vi "Build_Header_ARG.vi"(9 "All_Bundled_Data_Brass":T1, 10 "ERD Number Array In":string[](array[string]), 11 "ERD Name Array In":string[](array[string])) -> (2 "ERD Name Array out 2":string[][](array[string]))   [LabVIEW 2021]
uses:
  Type defs/All_Bundled_Data_ARG.ctl
  Dryer Tool (Commercial 2)/JL Dryer Tool Support/type defs/Version.ctl
  Dryer Tool (Commercial 2)/JL Dryer Tool Support/type defs/CSV_File_String_Arrays.ctl
  Dryer Tool (Commercial 2)/JL Dryer Tool Support/type defs/Fault Table Array.ctl
  Dryer Tool (Commercial 2)/JL Dryer Tool Support/type defs/Fault_Table_Info.ctl
  Dryer Tool (Commercial 2)/JL Dryer Tool Support/type defs/BootloaderVersion.ctl
  Type defs/ERD_Always_Show_ARG.ctl
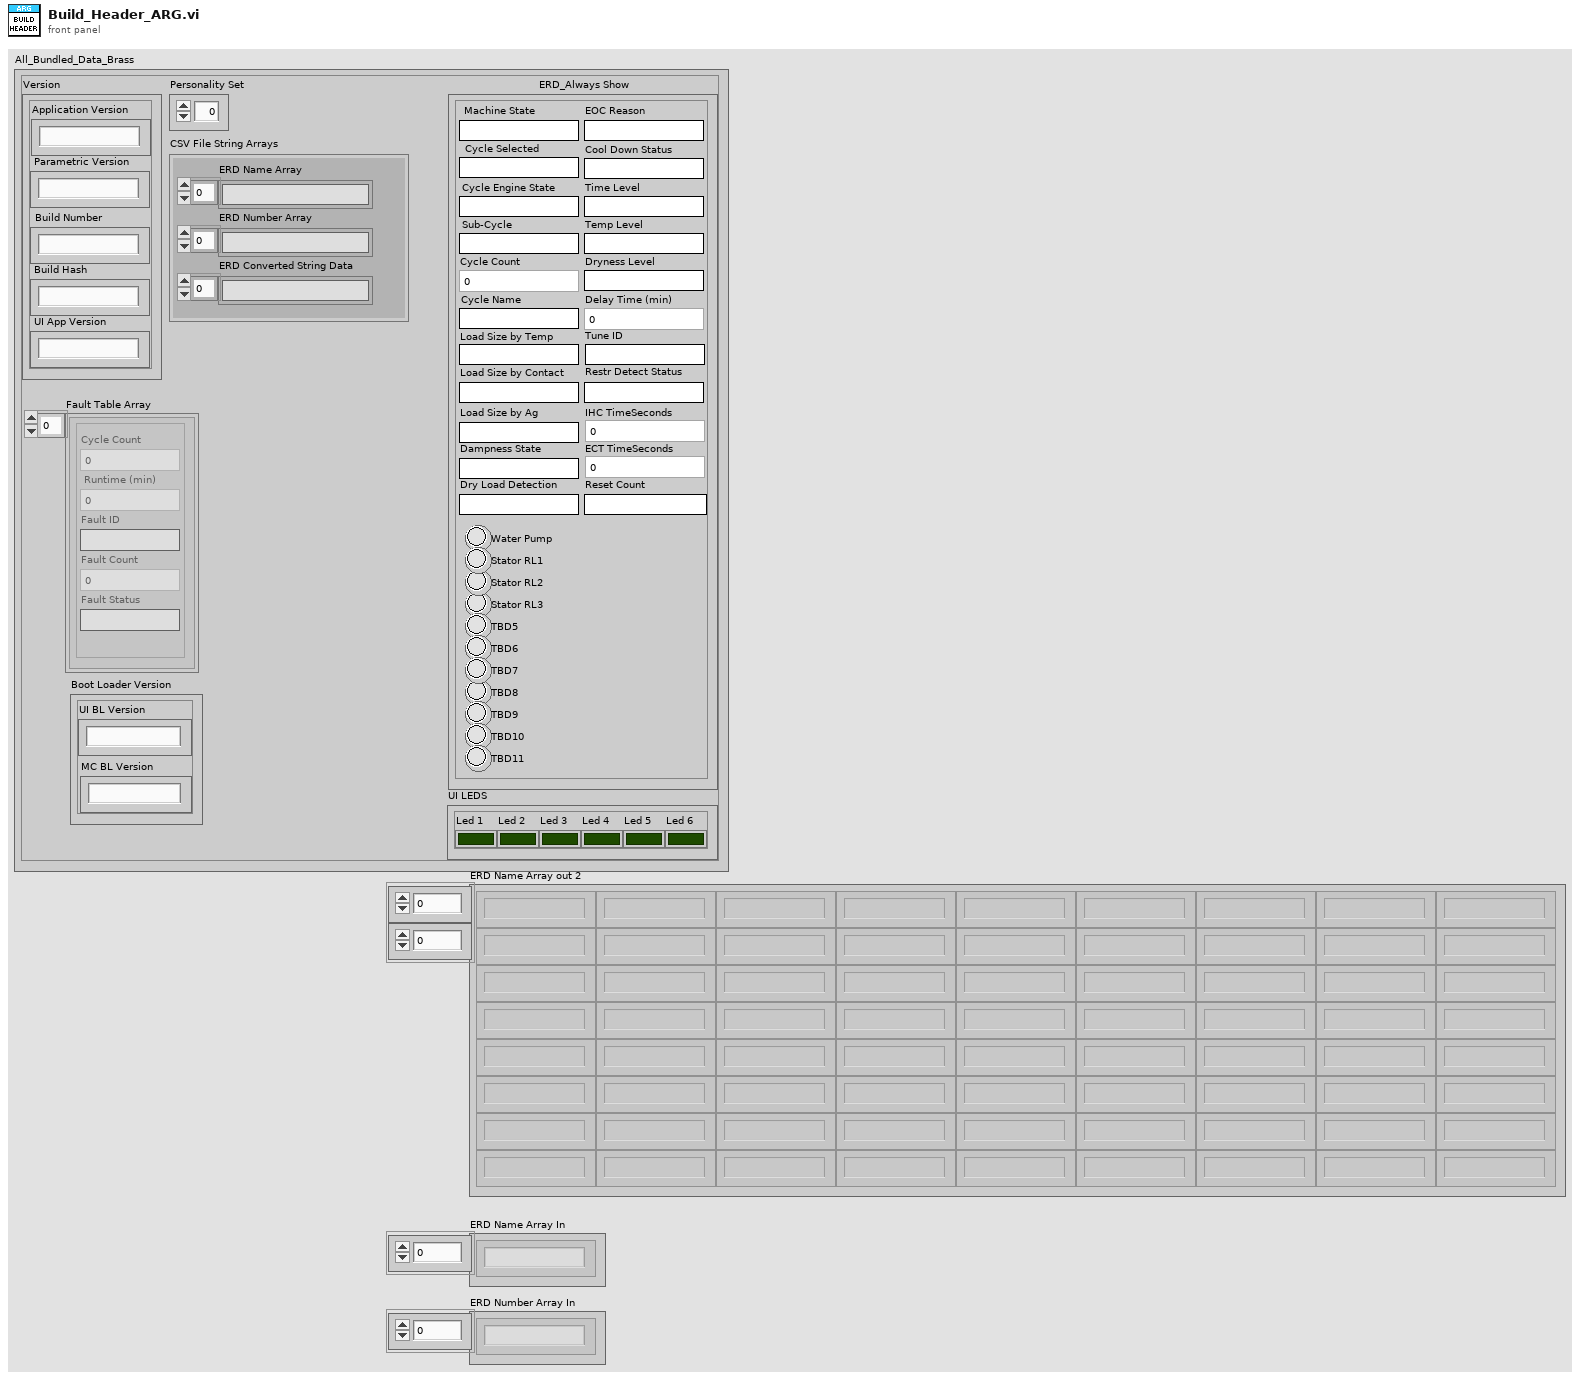
[diagram p1: front panel]
types:
  T1 = typedef "All_Bundled_Data_ARG.ctl" = cluster{"Version":T2, "Personality Set":u8, "CSV File String Arrays":T3, "Fault Table Array ":T4, "Boot Loader Version":T6, "ERD_Always Show":T7, "UI LEDS":cluster{"Led 1":bool, "Led 2":bool, "Led 3":bool, "Led 4":bool, "Led 5":bool, "Led 6":bool}}
  T2 = typedef "Version.ctl" = cluster{"Build Number":string, "Build Hash ":string, "Application Version":string, "Parametric Version":string, "UI App Version":string}
  T3 = typedef "CSV_File_String_Arrays.ctl" = cluster{"ERD Number Array":string[], "ERD Name Array":string[], "ERD Converted String Data":string[]}
  T4 = typedef "Fault Table Array.ctl" = T5[]
  T5 = typedef "Fault_Table_Info.ctl" = cluster{"Cycle Count":u32, " Runtime (min) ":u32, "Fault Status":string, "Fault ID":string, "Fault Count":u16}
  T6 = typedef "BootloaderVersion.ctl" = cluster{"UI BL Version":string, "MC BL Version":string}
  T7 = typedef "ERD_Always_Show_ARG.ctl" = cluster{"Machine State":string, "Cycle Selected":string, "Cycle Engine State":string, "Cycle Count":u32, "Temp Level":string, "Dryness Level":string, "Time Level":string, "Delay Time (min)":u16, "Sub-Cycle":string, "Cycle Name":string, "Tune ID":string, "Restr Detect Status":string, "Load Size by Contact":string, "Load Size by Temp":string, "EOC Reason":string, "Reset Count":string, "Dampness State":string, "Stator RL3":bool, "TBD5":bool, "TBD6":bool, "Water Pump":bool, "Stator RL2":bool, "Cool Down Status":string, "TBD8":bool, "TBD9":bool, "TBD10":bool, "TBD11":bool, "TBD7":bool, "Stator RL1":bool, "IHC TimeSeconds":u32, "ECT TimeSeconds ":u32, "Load Size by Ag":string, "Dry Load Detection":string}
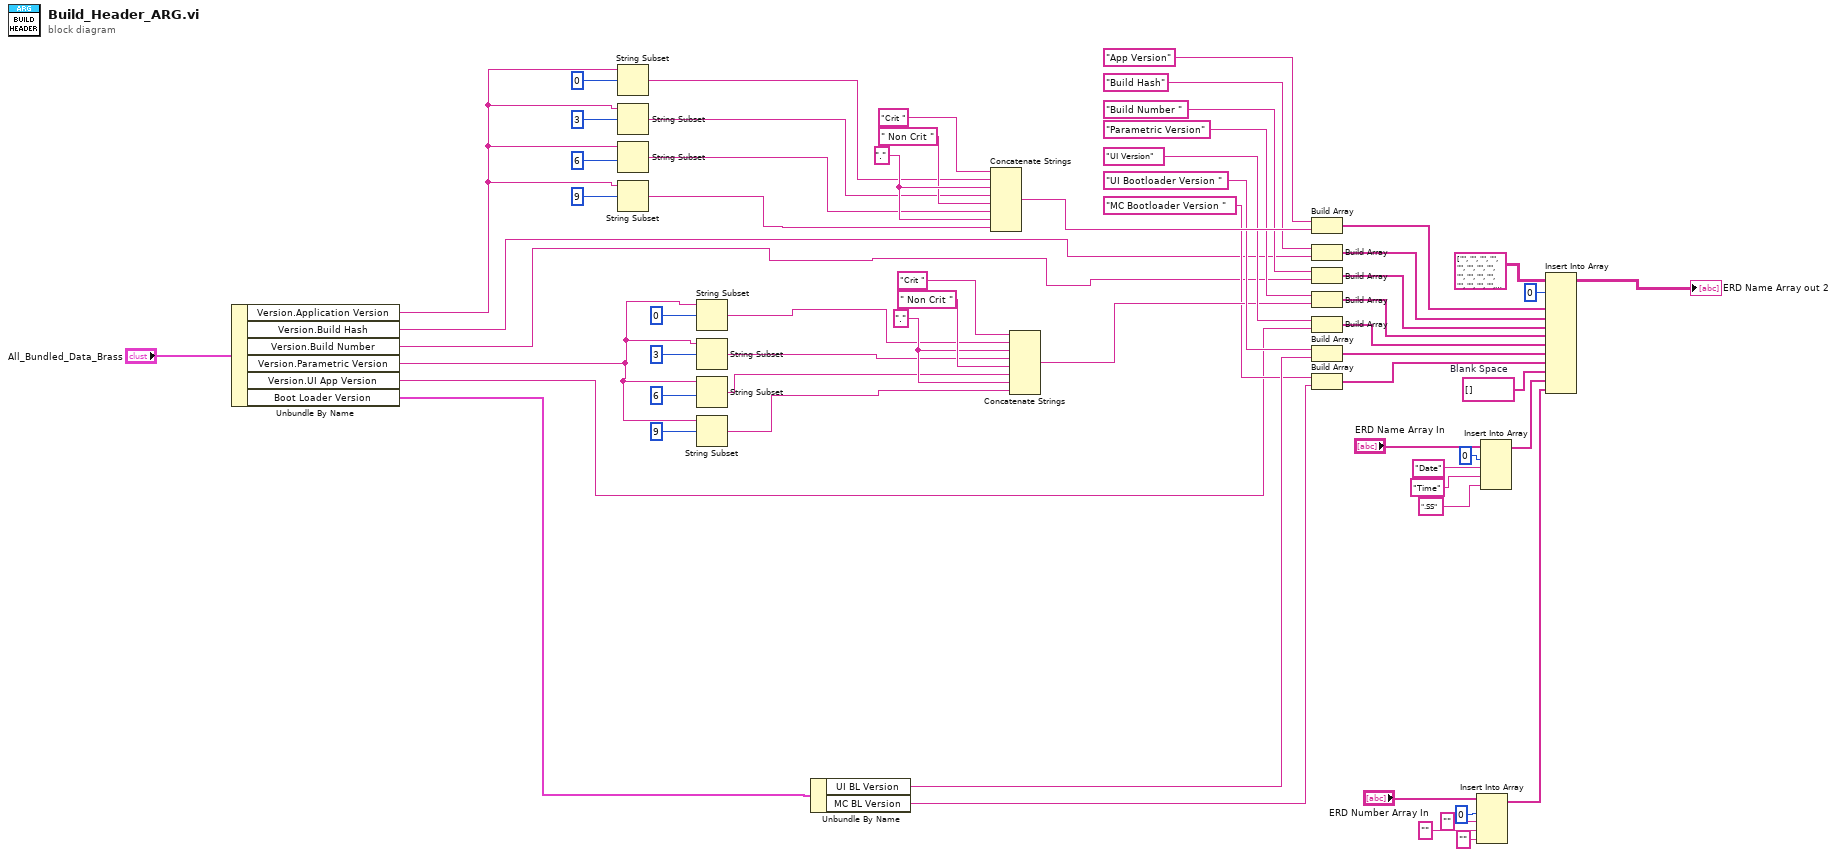
[diagram p0: block diagram]
diagram:
  w27 = string[] []  # Blank Space
  w58 = "." ("element")
  w63 = "." ("element")
  n1 = Unbundle By Name("All_Bundled_Data_Brass") -> ("Version.Application Version"=w19:string, "Version.Build Hash"=w10:string, "Version.Build Number"=w9:string, "Version.Parametric Version"=w8:string, "Version.UI App Version"=w3:string, "Boot Loader Version"=w2:T6)
  n2 = String Subset(string=w19, offset (0)=0 ("length (rest)")) -> (substring=w18:string)  [unwired: 1 in]
  n3 = String Subset(string=w19, offset (0)=3 ("length (rest)")) -> (substring=w17:string)  [unwired: 1 in]
  n4 = String Subset(string=w19, offset (0)=6) -> (substring=w16:string)  [unwired: 1 in]
  n5 = String Subset(string=w19, offset (0)=9) -> (substring=w15:string)  [unwired: 1 in]
  n6 = String Subset(string=w8, offset (0)=0 ("length (rest)")) -> (substring=w7:string)  [unwired: 1 in]
  n7 = String Subset(string=w8, offset (0)=3 ("length (rest)")) -> (substring=w6:string)  [unwired: 1 in]
  n8 = String Subset(string=w8, offset (0)=6) -> (substring=w5:string)  [unwired: 1 in]
  n9 = String Subset(string=w8, offset (0)=9) -> (substring=w4:string)  [unwired: 1 in]
  n10 = Unbundle By Name(w2) -> ("UI BL Version"=w38:string, "MC BL Version"=w28:string)
  n11 = Concatenate Strings("Crit " ("element"), w18, w63, w17, " Non Crit " ("element"), w16, w63, w15) -> (w54:string)
  n12 = Concatenate Strings("Crit " ("element"), w7, w58, w6, " Non Crit " ("element"), w5, w58, w4) -> (w37:string)
  n13 = Build Array("App Version" ("new element/subarray"), w54) -> (w56:string[])
  n14 = Build Array("Build Hash" ("new element/subarray"), w10) -> (w52:string[])
  n15 = Build Array("Build Number " ("new element/subarray"), w9) -> (w50:string[])
  n16 = Build Array("Parametric Version" ("new element/subarray"), w37) -> (w49:string[])
  n17 = Build Array("UI Version" ("new element/subarray"), w3) -> (w48:string[])
  n18 = Build Array("UI Bootloader Version " ("new element/subarray"), w38) -> (w36:string[])
  n19 = Build Array("MC Bootloader Version " ("new element/subarray"), w28) -> (w24:string[])
  n20 = Insert Into Array(array="ERD Number Array In", index=0, new element #1="" ("new element/subarray"), new element #2="" ("new element/subarray"), new element #3="" ("new element/subarray")) -> (w25:string[])
  n21 = Insert Into Array(array="ERD Name Array In", index=0, new element #1="Date", new element #2="Time", new element #3=".SS" ("new element/subarray")) -> (w26:string[])
  n22 = Insert Into Array(array=string[][] [["", "", "", "", "", "", "", "", "", "", "", "", "", "", "", "", "", "", "", "", "", "", "", "", "", "", "", "", "", "", "", "", "", "", "", "", "", "", "", "", "0"]] ("Array Ini"), index (row)=0, new element #1=w56, new element #2=w52, new element #3=w50, new element #4=w49, new element #5=w48, new element #6=w36, new element #7=w24, new element #8=w27, new element #9=w26, new element #10=w25) -> (→"ERD Name Array out 2":string[][])  [unwired: 1 in]
